vi "Write State.vi"(8 "error in (no error)":errorcluster, 10 "State":refnum<class "State Pattern.lvclass">, 11 "Context in":refnum<class "Context.lvclass">) -> (0 "error out":errorcluster, 3 "Context out":refnum<class "Context.lvclass">)   [LabVIEW 2021, in "Context.lvlib" / "Context.lvclass"]
uses:
  Context.lvclass
  State Pattern/State Pattern.lvclass
  Context State/Context State.lvclass
  Context.lvclass/Context.ctl
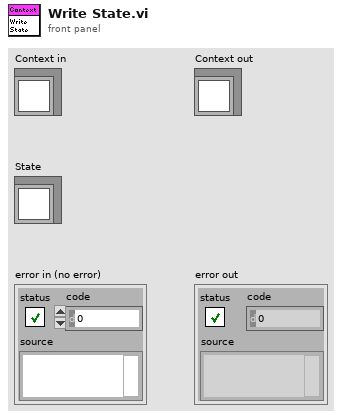
[diagram p1: front panel]
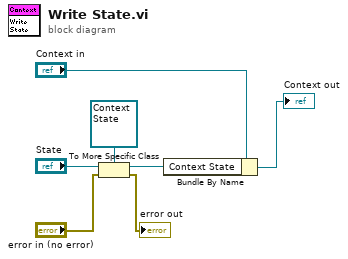
[diagram p0: block diagram]
diagram:
  n1 = To More Specific Class(target class=refnum<class "Context State.lvclass"> refnum ("Context.lvlib:Context State.lvclass"), reference="State", error in="error in (no error)") -> (specific class reference=w5:refnum<class "Context State.lvclass">, error out=→"error out":errorcluster)
  n2 = Bundle By Name(cluster="Context in", "Context State"=w5) -> (→"Context out":refnum<class "Context.lvclass">)
